vi "Binary Actor Example.vi"() -> ()   [LabVIEW 2019]
uses:
  ASCII/Actor/ASCII Actor.lvlib
  Binary Actor.lvlib
panel:
  out "Graph":dbl[](graph)
  in  "Number of Responses":i32
  in  "Request Data":bool
  out "Response":string
  in  "Send":bool
  in  "Message":string
  in  "VISA resource name":refnum<visa-resource-name>
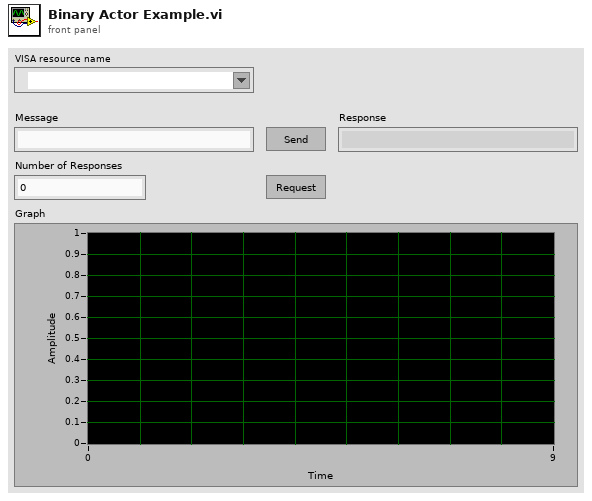
[diagram p1: front panel]
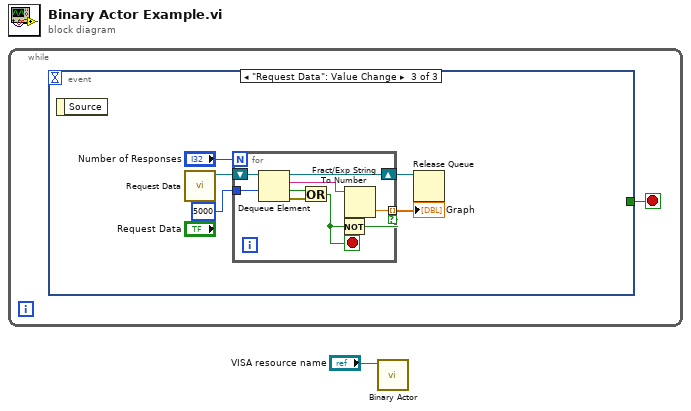
[diagram p0: block diagram]
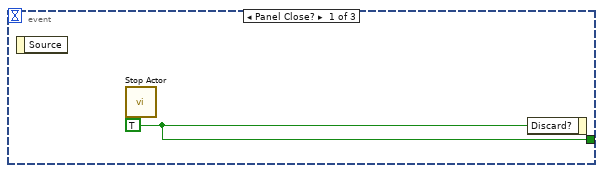
[diagram p2: hidden frame]
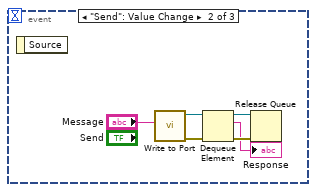
[diagram p3: hidden frame]
diagram:
  n1 = while {
    stop <- w2 stop-if-true
    n2 = event shown="[2] \"Request Data\": Value Change" {
      selector: _ -> [_ _ _]
      dyn-events: _ -> [_ _ _]
      timeout: _ -> [_ _ _]
      tunnel: [w3 _ _] -> w2
      event Panel Close? {
        w3 = TRUE ("Discard?")
        n3 = event-data() -> ()  [unwired: 1 in, 1 out]
        n4 = call "Stop Actor.vi"() -> ()  [unwired: 11 in, 1 out]
        n5 = event-data("Discard?"=w3) -> ()  [unwired: 1 in, 1 out]
      }
      event "Send": Value Change {
        n6 = event-data() -> ()  [unwired: 1 in, 1 out]
        n7 = call "Write to Port.vi"("Data"="Message") -> ("error out"=w9:errorcluster, "Response Queue"=w6:refnum<queue>)  [unwired: 9 in]
        n8 = Dequeue Element(queue=w6, error in (no error)=w9) -> (queue out=w5:refnum<queue>, element=→"Response":string, error out=w8:errorcluster)  [unwired: 1 in, 1 out]
        n9 = Release Queue(queue=w5, error in (no error)=w8) -> ()  [unwired: 1 in, 3 out]
      }
      event "Request Data": Value Change {
        n10 = event-data() -> ()  [unwired: 1 in, 1 out]
        n11 = call "Request Data.vi"() -> ("Response Queue"=w14:refnum<queue>)  [unwired: 10 in, 1 out]
        n12 = for {
          N: "Number of Responses" -> [_]
          shift-right: [w21] -> w11
          shift-left: w14 -> [w23]
          tunnel: [w20] -> w12 mode=indexing if=w19
          tunnel: 5000 ("timeout in ms (-1)") -> [w18]
          stop <- w15 stop-if-true
          n13 = Dequeue Element(queue=w23, timeout in ms (-1)=w18) -> (queue out=w21:refnum<queue>, element=w22:string, timed out?=w17:bool, error out=w16:errorcluster)  [unwired: 1 in]
          n14 = Or(x=w17, y=w16) -> (x .or. y?=w15:bool)
          n15 = Not(x=w15) -> (.not. x?=w19:bool)
          n16 = Fract/Exp String To Number(string=w22) -> (number=w20:dbl)  [unwired: 3 in, 1 out]
        }
        "Graph" <- w12
        n17 = Release Queue(queue=w11) -> ()  [unwired: 2 in, 3 out]
      }
    }
  }
  n18 = call "Binary Actor.vi"("VISA resource name"="VISA resource name") -> ()  [unwired: 10 in, 1 out]
